vi "Init.vi"(8 "error in (no error)":errorcluster, 10 "Settings":T1, 11 "Ramp Voltage In":refnum<class "Ramp Voltage.lvclass">) -> (0 "error out":errorcluster, 3 "Ramp Voltage Out":refnum<class "Ramp Voltage.lvclass">)   [LabVIEW 2020, in "High Level PSU With Tests.lvlib" / "Ramp Voltage.lvclass"]
uses:
  Ramp Voltage.lvclass
  Ramp Settings.ctl
  Ramp Voltage.lvclass/Ramp Voltage.ctl
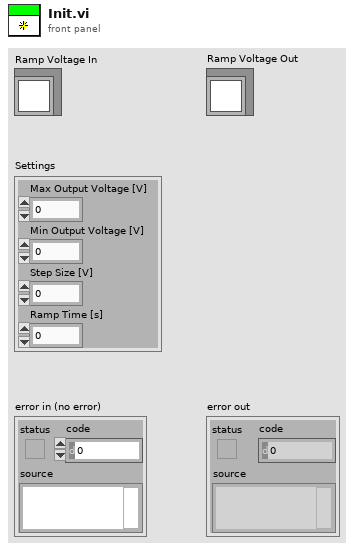
[diagram p1: front panel]
types:
  T1 = typedef "High Level PSU With Tests.lvlib/Ramp Voltage.lvclass/Ramp Settings.ctl" = cluster{"Max Output Voltage [V]":dbl, "Min Output Voltage [V]":dbl, "Step Size [V]":dbl, "Ramp Time [s]":dbl}
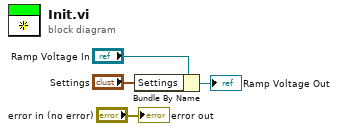
[diagram p0: block diagram]
diagram:
  n1 = Bundle By Name(cluster="Ramp Voltage In", "Settings"="Settings") -> (→"Ramp Voltage Out":refnum<class "Ramp Voltage.lvclass">)
  "error out" <- "error in (no error)"
